vi "build table.vi"(8 "error in (no error)":errorcluster, 10 "Sort Types":string[](array[string]), 11 "resource table in":string[][](array[string])) -> (0 "error out":errorcluster, 1 "max string length in columns":i32[](array[numeric]), 2 "Headers":string[](array[string]), 3 "resource table out":string[][](array[string]))   [LabVIEW 2016, in "FPGA RM System Definition API.lvlib"]
uses:
  FPGA-Resource-Manager-APIs/Source/System Definition/FPGA RM System Definition API.lvlib
  visualizer globals.vi
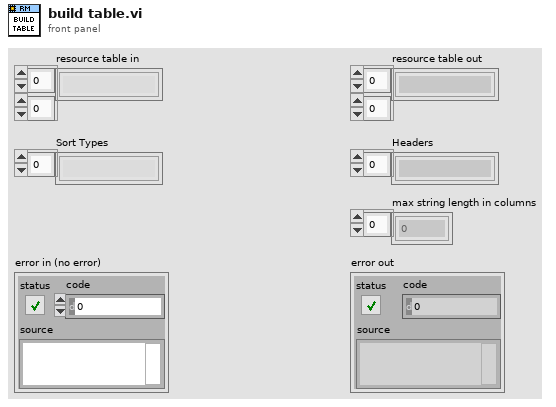
[diagram p1: front panel]
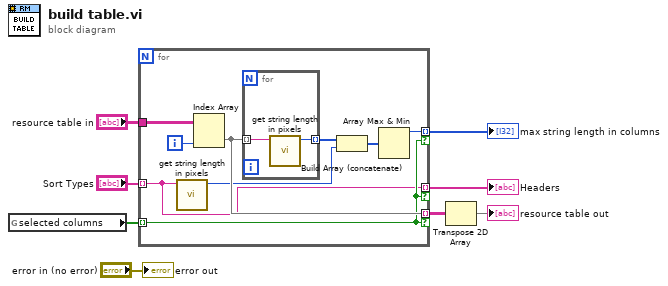
[diagram p0: block diagram]
diagram:
  n1 = global read "visualizer globals.vi" "selected columns"() -> (w1:bool[])
  n2 = for {
    tunnel: w1 -> [w11] mode=indexing
    tunnel: "Sort Types" -> [w10] mode=indexing
    tunnel: [w10] -> w6 mode=indexing if=w11
    tunnel: [w15] -> w7 mode=indexing if=w11
    tunnel: "resource table in" -> [w17]
    tunnel: [w14] -> w2 mode=indexing if=w11
    i -> [w16]
    n3 = call "get string length in pixels.vi"("notes"=w10) -> ("Numeric"=w9:i16)  [unwired: 10 in]
    n4 = Index Array(array=w17, index (col)=w16) -> (element=w15:string[])  [unwired: 1 in]
    n5 = for {
      tunnel: w15 -> [w19] mode=indexing
      tunnel: [w18] -> w13 mode=indexing
      n6 = call "get string length in pixels.vi"("notes"=w19) -> ("Numeric"=w18:i16)  [unwired: 10 in]
    }
    n7 = Build Array (concatenate)(w13, w9) -> (w12:i16[])
    n8 = Array Max & Min(array=w12) -> (max value=w14:i16)  [unwired: 3 out]
  }
  "Headers" <- w6
  "max string length in columns" <- w2
  n9 = Transpose 2D Array(2D array=w7) -> (transposed array=→"resource table out":string[][])
  "error out" <- "error in (no error)"
